vi "MF-101 Counter Timer - PWM with measure pulse width.vi"() -> ()   [LabVIEW 8.6]
uses:
  vi.lib/UeiDaq/UeiDaqConfigureTimingForSimpleIO.vi
  <libdir>/resource/objmgr/ueidaq.rc
  vi.lib/UeiDaq/UeiDaqReadOneCounterScanUInt32.vi
  vi.lib/UeiDaq/UeiDaqCreateDIIndustrialSession.vi
  vi.lib/UeiDaq/UeiDaqCreateCISession.vi
  vi.lib/UeiDaq/UeiDaqCreateCOSession.vi
panel:
  out "Tick 2 (high) ms":dbl
  out "Tick1 (low) ms":dbl
  in  "High Threshold":dbl
  in  "Low Threshold":dbl
  in  "Digital resource":string
  out "pulse width":u32
  in  "Tick 2 (high)":i32
  in  "Tick1 (low)":i32
  in  "number of pulses to generate":i32
  in  "Input resource":string
  in  "Output resource":string
  in  "Refresh rate (ms)":u32
  in  "stop":bool
  # "MF-101 PWM with measure pulse width"
  # "need voltage on the appropriate DV pins for this example to work"
  # "There are 2 available counter modules on the MF-101.  So no channels beyond 0, 1\ncan be used in the resource string.  Set source pin using ChannelList.CI.SourcePin and set output pin(s) using ChannelList.CO.OutputPins."
  # "Sampling frequency for Guardian is 400kHz for resolution of 2.5usec"
  # "__"
  # "1 tick = 1/66,000,000 = 1.515151e-8"
  # "(66Mhz clock)"
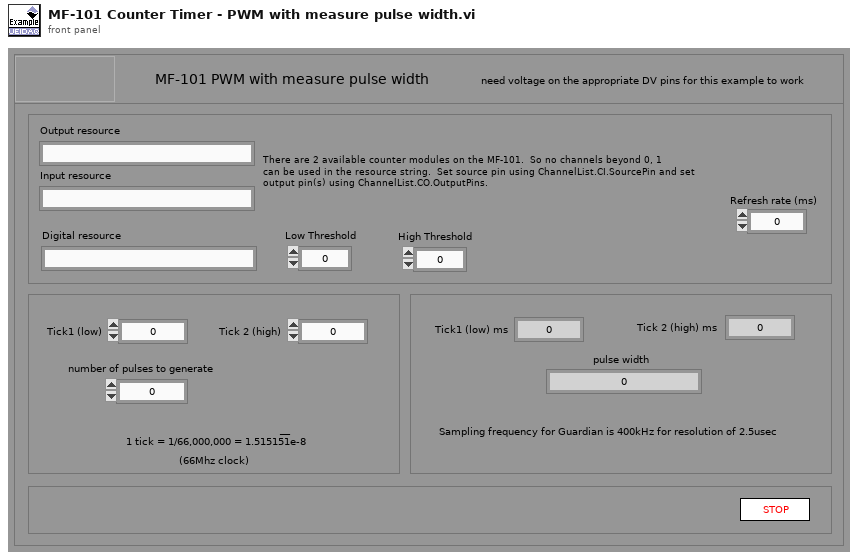
[diagram p1: front panel]
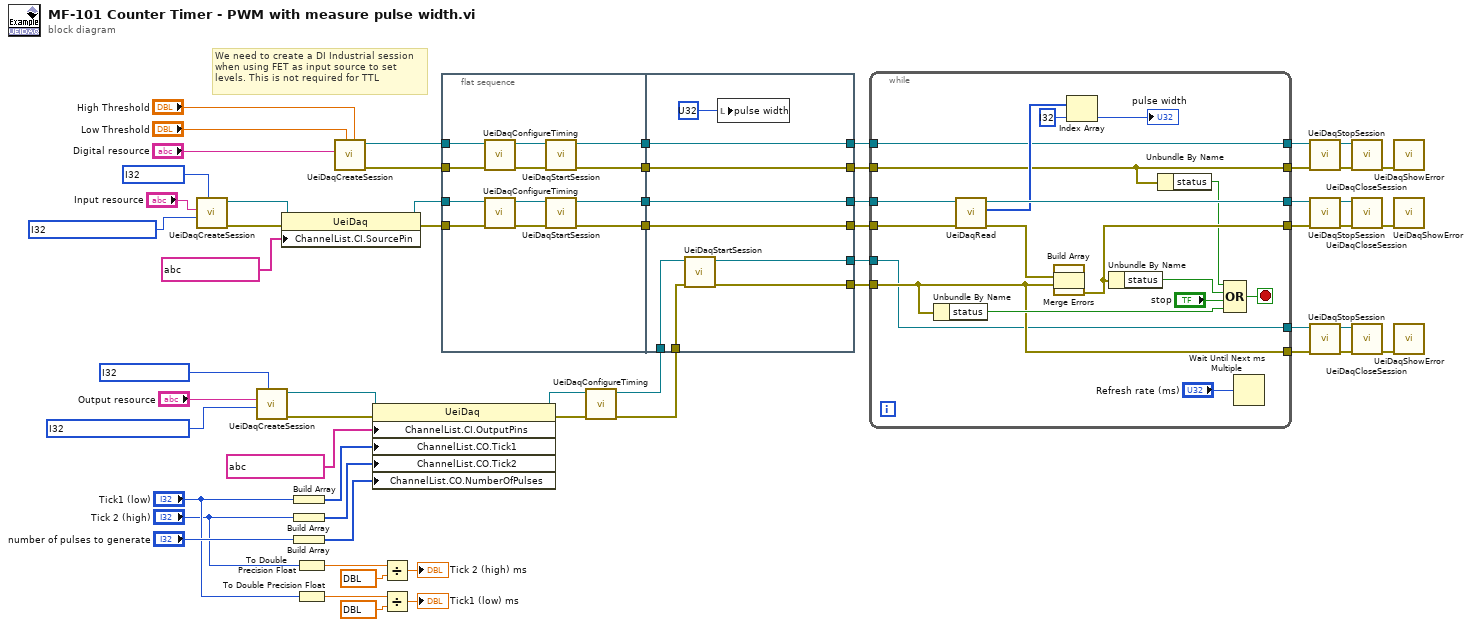
[diagram p0: block diagram]
diagram:
  w54 = i32 ? items=["Count Events", "Measure Pulse Width", "Measure Period", "Generate Pulse", "Generate Pulse Train", "Pulse width modulation", "Quadrature encoder"] ("Counter Mode")
  w55 = i32 ? items=["Internal Clock", "Internal Clock divided by 2", "External ", "Counter 0 Output", "Counter 1 Output", "Counter 2 Output"] ("Counter Source")
  w57 = i32 ? items=["Count Events", "Measure Pulse Width", "Measure Period", "Generate Pulse", "Generate Pulse Train", "Pulse width modulation", "Quadrature encoder"] ("Counter Mode")
  w58 = i32 ? items=["Internal Clock", "Internal Clock divided by 2", "External ", "Counter 0 Output", "Counter 1 Output", "Counter 2 Output"] ("Counter Source")
  # "We need to create a DI Industrial session\nwhen using FET as input source to set\nlevels. This is not required for TTL"
  n1 = call-poly "UeiDaqCreateSession.vi"("Counter Source"=w55, "Counter Mode"=w54, "Resource"="Input resource") -> ("error out"=w46:errorcluster, "UeiDaq Refnum Out"=w48:refnum<k20>)  [unwired: 5 in, 2 out]
  n2 = call-poly "UeiDaqCreateSession.vi"("Counter Source"=w58, "Counter Mode"=w57, "Resource"="Output resource") -> ("error out"=w51:errorcluster, "UeiDaq Refnum Out"=w52:refnum<k20>)  [unwired: 6 in, 1 out]
  n3 = property class="UeiDaq"(reference=w48, error in=w46, "ChannelList.CI.SourcePin"=string[] ? ("Channel List:Counter Output:Output Pins")) -> (reference out=w47:refnum<k20>, error out=w45:errorcluster)
  n4 = Build Array("Tick1 (low)") -> (w32:i32[])
  n5 = Build Array("Tick 2 (high)") -> (w41:i32[])
  n6 = Build Array("number of pulses to generate") -> (w40:i32[])
  n7 = To Double Precision Float(number="Tick 2 (high)") -> (double precision float=w44:dbl)
  n8 = To Double Precision Float(number="Tick1 (low)") -> (double precision float=w16:dbl)
  n9 = call-poly "UeiDaqCreateSession.vi"("High Threshold"="High Threshold", "Low Threshold"="Low Threshold", "Resource"="Digital resource") -> ("error out"=w27:errorcluster, "UeiDaq Refnum Out"=w28:refnum<k20>)  [unwired: 7 in]
  n10 = property class="UeiDaq"(reference=w52, error in=w51, "ChannelList.CI.OutputPins"=string[] ? ("Channel List:Counter Output:Output Pins"), "ChannelList.CO.Tick1"=w32, "ChannelList.CO.Tick2"=w41, "ChannelList.CO.NumberOfPulses"=w40) -> (reference out=w50:refnum<k20>, error out=w49:errorcluster)
  n11 = Divide(x=w44, y=dbl ?) -> (x/y=→"Tick 2 (high) ms":dbl)
  n12 = Divide(x=w16, y=dbl ?) -> (x/y=→"Tick1 (low) ms":dbl)
  n13 = flat-sequence {
    tunnel: w47 -> [w68]
    tunnel: w45 -> [w67]
    tunnel: w28 -> [w66]
    tunnel: w27 -> [w65]
    tunnel: [w70] -> w12
    tunnel: [w69] -> w11
    tunnel: [w62] -> w10
    tunnel: [w61] -> w9
    tunnel: [w80] -> w24
    tunnel: [w81] -> w25
    tunnel: [w74] -> w13
    tunnel: w9 -> [w80]
    tunnel: w10 -> [w81]
    tunnel: w11 -> [w78]
    tunnel: w12 -> [w79]
    tunnel: [w79] -> w6
    tunnel: [w78] -> w5
    tunnel: w4 -> [w77]
    tunnel: w3 -> [w76]
    tunnel: [w73] -> w1
    frame #0 {
      n14 = call-poly "UeiDaqConfigureTiming.vi"("error in (no error)"=w65, "UeiDaq Refnum In"=w66) -> ("error out"=w63:errorcluster, "UeiDaq Refnum Out"=w64:refnum<k20>)  [unwired: 1 in, 7 out]
      n15 = call-poly "UeiDaqConfigureTiming.vi"("error in (no error)"=w67, "UeiDaq Refnum In"=w68) -> ("error out"=w71:errorcluster, "UeiDaq Refnum Out"=w72:refnum<k20>)  [unwired: 1 in, 7 out]
      n16 = call "UeiDaqStartSession.vi"("error in (no error)"=w63, "UeiDaq Refnum In"=w64) -> ("error out"=w61:errorcluster, "UeiDaq Refnum Out"=w62:refnum<k20>)  [unwired: 8 out]
      n17 = call "UeiDaqStartSession.vi"("error in (no error)"=w71, "UeiDaq Refnum In"=w72) -> ("error out"=w69:errorcluster, "UeiDaq Refnum Out"=w70:refnum<k20>)  [unwired: 8 out]
    }
    frame #1 {
      n18 = call "UeiDaqStartSession.vi"("error in (no error)"=w77, "UeiDaq Refnum In"=w76) -> ("error out"=w74:errorcluster, "UeiDaq Refnum Out"=w73:refnum<k20>)  [unwired: 8 out]
      n19 = local write "pulse width"(u32 ? ("number of pulses")) -> ()
    }
  }
  n20 = call-poly "UeiDaqConfigureTiming.vi"("error in (no error)"=w49, "UeiDaq Refnum In"=w50) -> ("error out"=w4:errorcluster, "UeiDaq Refnum Out"=w3:refnum<k20>)  [unwired: 1 in, 7 out]
  n21 = while {
    tunnel: [w100] -> w37
    tunnel: w25 -> [w89]
    tunnel: w24 -> [w88]
    tunnel: [w88] -> w20
    tunnel: [w89] -> w19
    tunnel: w13 -> [w85]
    tunnel: [w83] -> w8
    tunnel: [w85] -> w7
    tunnel: w6 -> [w84]
    tunnel: w5 -> [w95]
    tunnel: [w93] -> w39
    tunnel: w1 -> [w83]
    stop <- w97 stop-if-true
    n22 = Unbundle By Name(w85) -> ("status"=w86:bool)
    n23 = call-poly "UeiDaqRead.vi"("error in (no error)"=w95, "UeiDaq Refnum In"=w84) -> ("error out"=w94:errorcluster, "Raw Data"=w92:u32[], "UeiDaq Refnum Out"=w100:refnum<k20>)  [unwired: 7 out]
    n24 = Build Array(w94, w85) -> (w82:errorcluster[])
    n25 = call <vilib>:"Merge Errors.vi"("error array in"=w82) -> ("error out"=w93:errorcluster)  [unwired: 6 in]
    n26 = Index Array(array=w92, index=i32 ?) -> (element=→"pulse width":u32)
    n27 = Unbundle By Name(w93) -> ("status"=w99:bool)
    n28 = Unbundle By Name(w88) -> ("status"=w87:bool)
    n29 = Compound Arithmetic op=OR(w87, w99, "stop", w86) -> (w97:bool)
    n30 = Wait Until Next ms Multiple(millisecond multiple="Refresh rate (ms)") -> ()  [unwired: 1 out]
  }
  n31 = call "UeiDaqStopSession.vi"("error in (no error)"=w20, "UeiDaq Refnum In"=w19) -> ("error out"=w22:errorcluster, "UeiDaq Refnum Out"=w23:refnum<k20>)  [unwired: 8 in]
  n32 = call "UeiDaqStopSession.vi"("error in (no error)"=w39, "UeiDaq Refnum In"=w37) -> ("error out"=w38:errorcluster, "UeiDaq Refnum Out"=w36:refnum<k20>)  [unwired: 8 in]
  n33 = call "UeiDaqStopSession.vi"("error in (no error)"=w7, "UeiDaq Refnum In"=w8) -> ("error out"=w35:errorcluster, "UeiDaq Refnum Out"=w34:refnum<k20>)  [unwired: 8 in]
  n34 = call "UeiDaqCloseSession.vi"("error in (no error)"=w22, "UeiDaq Refnum In"=w23) -> ("error out"=w21:errorcluster)  [unwired: 1 in, 8 out]
  n35 = call "UeiDaqCloseSession.vi"("error in (no error)"=w38, "UeiDaq Refnum In"=w36) -> ("error out"=w53:errorcluster)  [unwired: 1 in, 8 out]
  n36 = call "UeiDaqCloseSession.vi"("error in (no error)"=w35, "UeiDaq Refnum In"=w34) -> ("error out"=w60:errorcluster)  [unwired: 1 in, 8 out]
  n37 = call "UeiDaqShowError.vi"("error in (no error)"=w21) -> ()  [unwired: 2 in, 9 out]
  n38 = call "UeiDaqShowError.vi"("error in (no error)"=w53) -> ()  [unwired: 2 in, 9 out]
  n39 = call "UeiDaqShowError.vi"("error in (no error)"=w60) -> ()  [unwired: 2 in, 9 out]
